vi "Automatic operation loop.vi"() -> ()   [LabVIEW 2016]
uses:
  <userlib>/LevyLab/Relay Box/Type_defs/Resistor--enum.ctl
  <userlib>/LevyLab/General AFM Lithography/subVIs/Global Variables.vi
panel:
  in  "Pulse Settings":T2={"Z Set point"=-0.03, "Set Resistance"=enum."0 ohms", "Wait between"=0, "Withdraw tip? 1"=TRUE, "Set Resistance 2"=enum."0 ohms", "Withdraw tip? 2"=TRUE} {"Z Set point" format="%#_6p"}
  in  "Repeat pulses (set V1 type to be repeating)":dbl=10.0
  in  "Stop Button":bool
  in  "Ready to apply pulses ?":bool
  out "Next T2":dbl=1000.0
  out "Next V2":dbl=10.0
  out "Next T1":dbl=600.0
  out "Next V1":dbl=-13.0
  out "error out":errorcluster
  in  "Cluster":T3={"V2 array"=[0.0, 1.0, 2.0, 3.0, 4.0, 5.0], "V1 array"=[0.0, 1.0, 2.0, 3.0, 4.0, 5.0], "T2 array"=[4.0], "T1 array"=[4.0]}
  in  "First voltage pulse":T4={"Vmin"=0.0, "Tmin"=200.0, "Vmax"=5.0, "Tmax"=600.0, "V Array"=[0.0, 1.0, 1.0, 1.0, 1.0], "T Array"=[10.0, 20.0, 40.0, 60.0, 80.0, 100.0, 200.0, 300.0, 400.0, 500.0, 600.0], "V step"=1.0, "T step"=100.0, "Constant V"=-13.0, "Constant T"=600.0, "V1 type"=enum."No-Sweep", "T1 type"=enum."No-Sweep"}
  out "V1 array":dbl[](array[numeric])=[-13.0]
  out "T1 array":dbl[](array[numeric])=[600.0]
  in  "vi path":path=path "C:/Program Files (x86)/National Instruments/LabVIEW 2016/user.lib/LevyLab/General AFM Lithography/Main_v4.vi"
  out "vi running ?":bool
  in  "error in (no error)":errorcluster
  in  "Objects to enable":string[](array[string])=["r3", "p0", "p3"]
  out "T2 array":dbl[](array[numeric])=[200.0, 300.0, 400.0, 500.0, 600.0, 700.0, 800.0, 900.0, 1000.0]
  out "V2 array":dbl[](array[numeric])=[10.0]
  out "Log":string="Log:\nPulse: (-13.00V, 600.00ms); wait 5000ms; Pulse: (10V, 200ms), wait 10000ms is DONE\nPulse: (-13.00V, 600.00ms); wait 5000ms; Pulse: (10V, 300ms), wait 10000ms is DONE\nPulse: (-13.00V, 600.00ms); wait 5000ms; Pulse: (10V, 400ms), wait 10000ms is DONE\nPulse: (-13.00V, 600.00ms); wait 5000ms; Pulse: (10V, 500ms), wait 10000ms is DONE\nPulse: (-13.00V, 600.00ms); wait 5000ms; Pulse: (10V, 600ms), wait 10000ms is DONE\nPulse: (-13.00V, 600.00ms); wait 5000ms; Pulse: (10V, 700ms), wait 10000ms is DONE\nPulse: (-13.00V, 600.00ms); wait 5000ms; Pulse: (10V, 800ms), wait 10000ms is DONE\nPulse: (-13.00V, 600.00ms); wait 5000ms; Pulse: (10V, 900ms), wait 10000ms is DONE\nPulse: (-13.00V, 600.00ms); wait 5000ms; Pulse: (10V, 1000ms), wait 10000ms is DONE\n"
  in  "Operation loop":T5(array[cluster])=[{"String"="p1", "Enum"=enum."Object", "Wait after"=0.0}, {"String"=".001", "Enum"=enum."Object", "Wait after"=0.0}, {"String"="p2", "Enum"=enum."Object", "Wait after"=500.0}, {"String"="", "Enum"=enum."Voltage pulse", "Wait after"=500.0}, {"String"="", "Enum"=enum."IV measurement", "Wait after"=500.0}]
  in  "Second voltage pulse":T6={"Vmin"=0.0, "Tmin"=200.0, "Vmax"=5.0, "Tmax"=1000.0, "V Array"=[0.0, 1.0, 1.0, 1.0, 1.0], "T Array"=[3.0, 3.0, 3.0, 3.0, 3.0], "V step"=1.0, "T step"=100.0, "Constant V"=10.0, "Constant T"=0.0, "V2 type"=enum."No-Sweep", "T2 type"=enum."Sweep (auto)"}
  # "Show the log of voltage parameter setting and corresponding IV record file name"
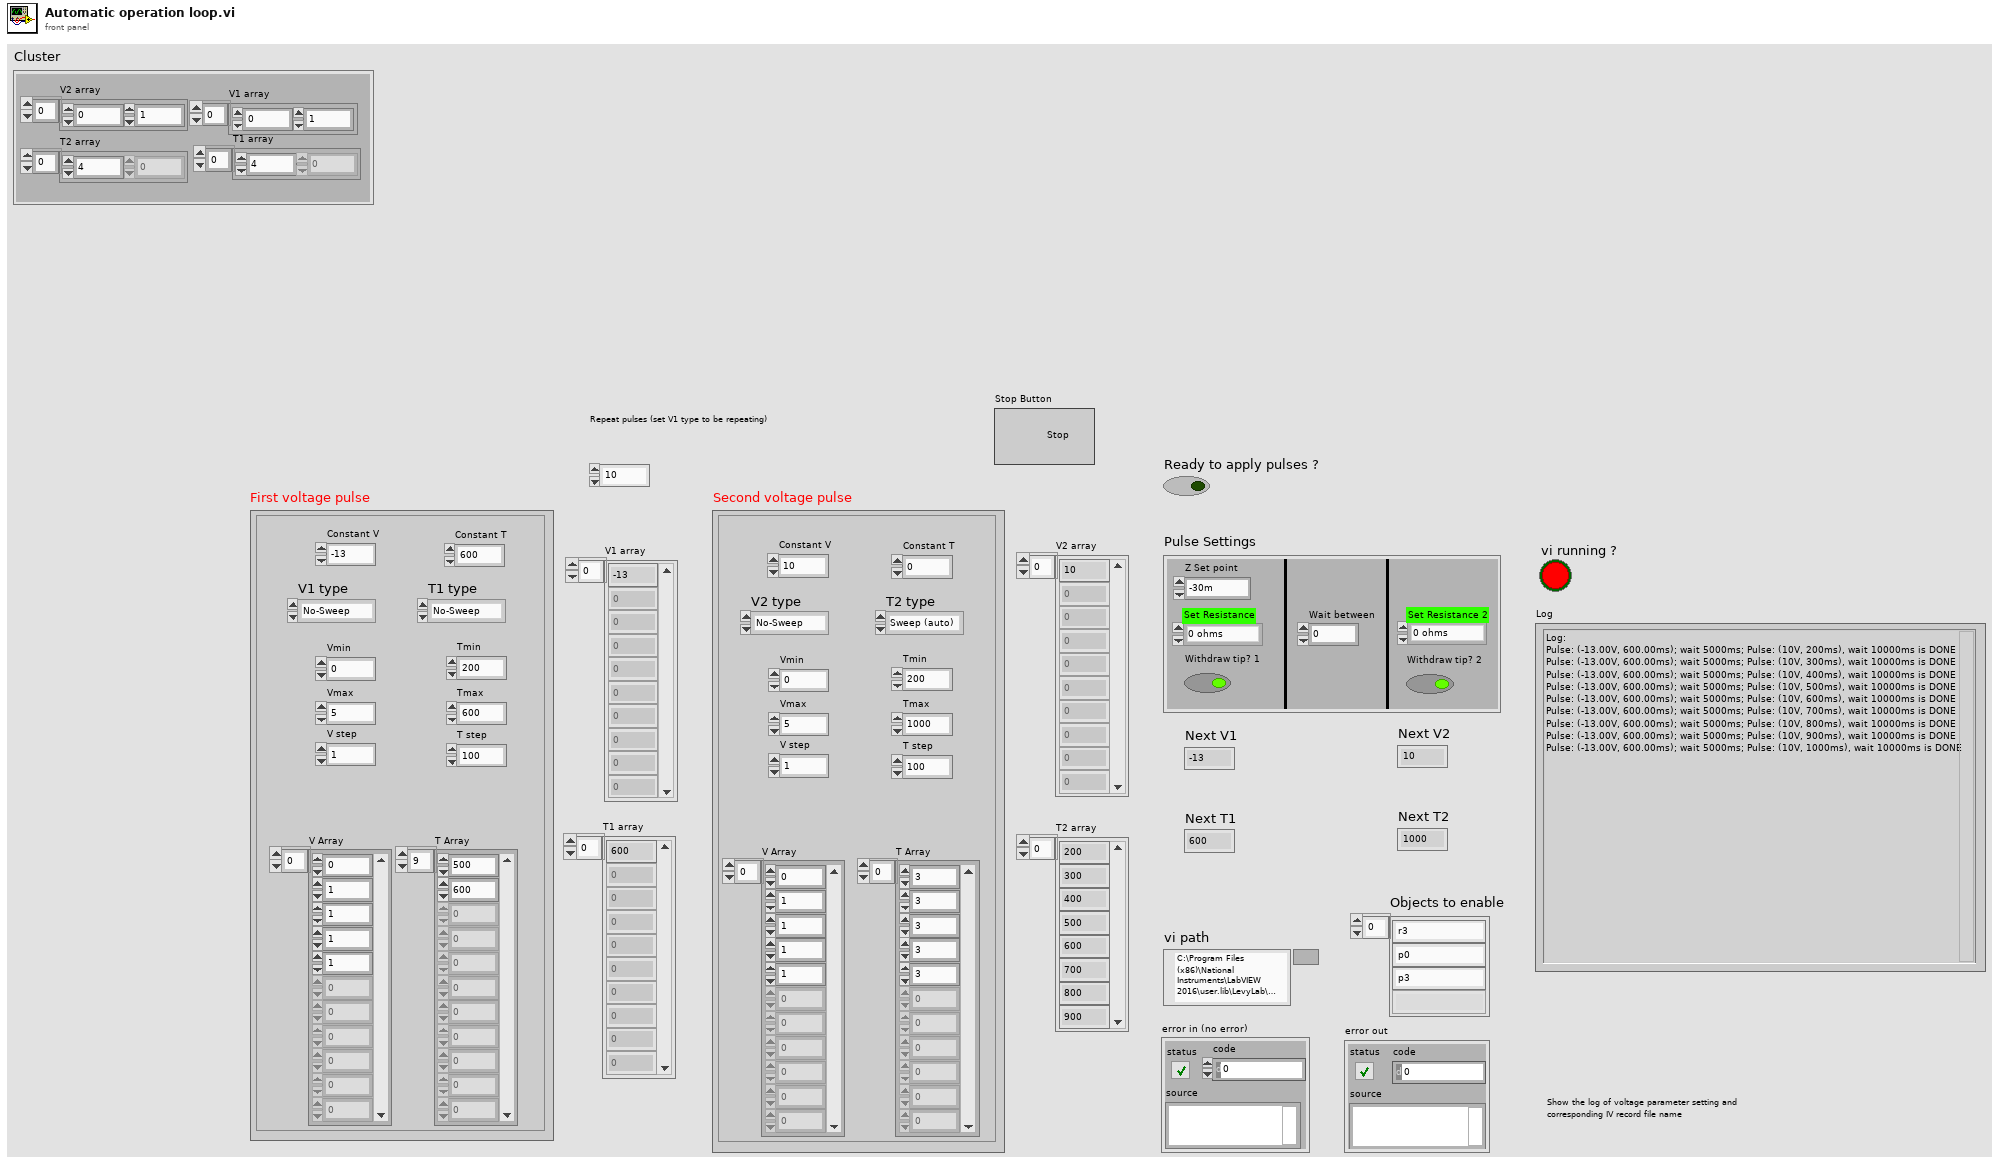
[diagram p1: front panel]
types:
  T1 = typedef "Resistor--enum.ctl" = enum16{"open", "discharge tip", "0 ohms", "100k ohm", "10M ohm", "1G ohm"}
  T2 = cluster{"Z Set point":dbl, "Set Resistance":T1, "Wait between":u32, "Withdraw tip? 1":bool, "Set Resistance 2":T1, "Withdraw tip? 2":bool}
  T3 = cluster{"V2 array":dbl[], "V1 array":dbl[], "T2 array":dbl[], "T1 array":dbl[]}
  T4 = cluster{"Vmin":dbl, "Tmin":dbl, "Vmax":dbl, "Tmax":dbl, "V Array":dbl[], "T Array":dbl[], "V step":dbl, "T step":dbl, "Constant V":dbl, "Constant T":dbl, "V1 type":enum16{"Repeating", "No-Sweep", "Sweep (manual)", "Sweep (auto)"}, "T1 type":enum16{"Repeating", "No-Sweep", "Sweep (manual)", "Sweep (auto)"}}
  T5 = cluster{"String":string, "Enum":enum16{"Object", "Voltage pulse", "IV measurement", "Change interpolation distance"}, "Wait after":dbl}[]
  T6 = cluster{"Vmin":dbl, "Tmin":dbl, "Vmax":dbl, "Tmax":dbl, "V Array":dbl[], "T Array":dbl[], "V step":dbl, "T step":dbl, "Constant V":dbl, "Constant T":dbl, "V2 type":enum16{"Repeating", "No-Sweep", "Sweep (manual)", "Sweep (auto)"}, "T2 type":enum16{"Repeating", "No-Sweep", "Sweep (manual)", "Sweep (auto)"}}
  T7 = enum16{"Object", "Voltage pulse", "IV measurement", "Change interpolation distance"}
  T8 = typedef "Funnel Properties - cluster.ctl" = cluster{"Enabled":bool, "Direction":u16, "Smooth Segments":dbl, "Bottom Segs.":dbl, "Speed (um/s)":T9, "Voltage (V)":T9, "Set Resistance":T1}
  T9 = typedef "Voltage - cluster.ctl" = cluster{"Schedule":T10, "Value":dbl, "Start Value":dbl, "End Value":dbl, "Min Value":dbl, "Max Value":dbl, "Duty Cycle (%)":dbl, "Signal Type":T11, "Cycle Number":dbl, "Phase (degrees)":dbl, "formula":string, "formula length (nm)":dbl, "formula resolution (nm)":dbl}
  T10 = typedef "Schedule - enum.ctl" = enum16{"Constant", "Ramp", "Fn. Generator", "Formula"}
  T11 = typedef "Signal Type - enum.ctl" = enum16{"Sine Wave", "Triangle Wave", "Square Wave", "Sawtooth Wave"}
  T12 = typedef "Path Properties - cluster.ctl" = cluster{"Enabled":bool, "Direction":u16, "Fill Orientation":u16, "Smooth Segments":dbl, "Fill Spacing":dbl, "Speed (um/s)":T9, "Voltage (V)":T9, "Set Resistance":T1}
  T13 = typedef "Rectangle Properties - cluster.ctl" = cluster{"Enabled":bool, "Direction":u16, "Fill Orientation":u16, "Fill Spacing":dbl, "Speed (um/s)":T9, "Voltage (V)":T9, "Set Resistance":T1}
  T14 = enum16{"Repeating", "No-Sweep", "Sweep (manual)", "Sweep (auto)"}
  T15 = cluster{"Set point":dbl, "Set Resistance":T1, "First pulse voltage":dbl, "First pulse time":u32, "Wait between":u32, "Second pulse voltage":dbl, "Second pulse time":u32, "Withdraw tip? 1":bool, "Set Resistance 2":T1, "Withdraw tip? 2":bool}
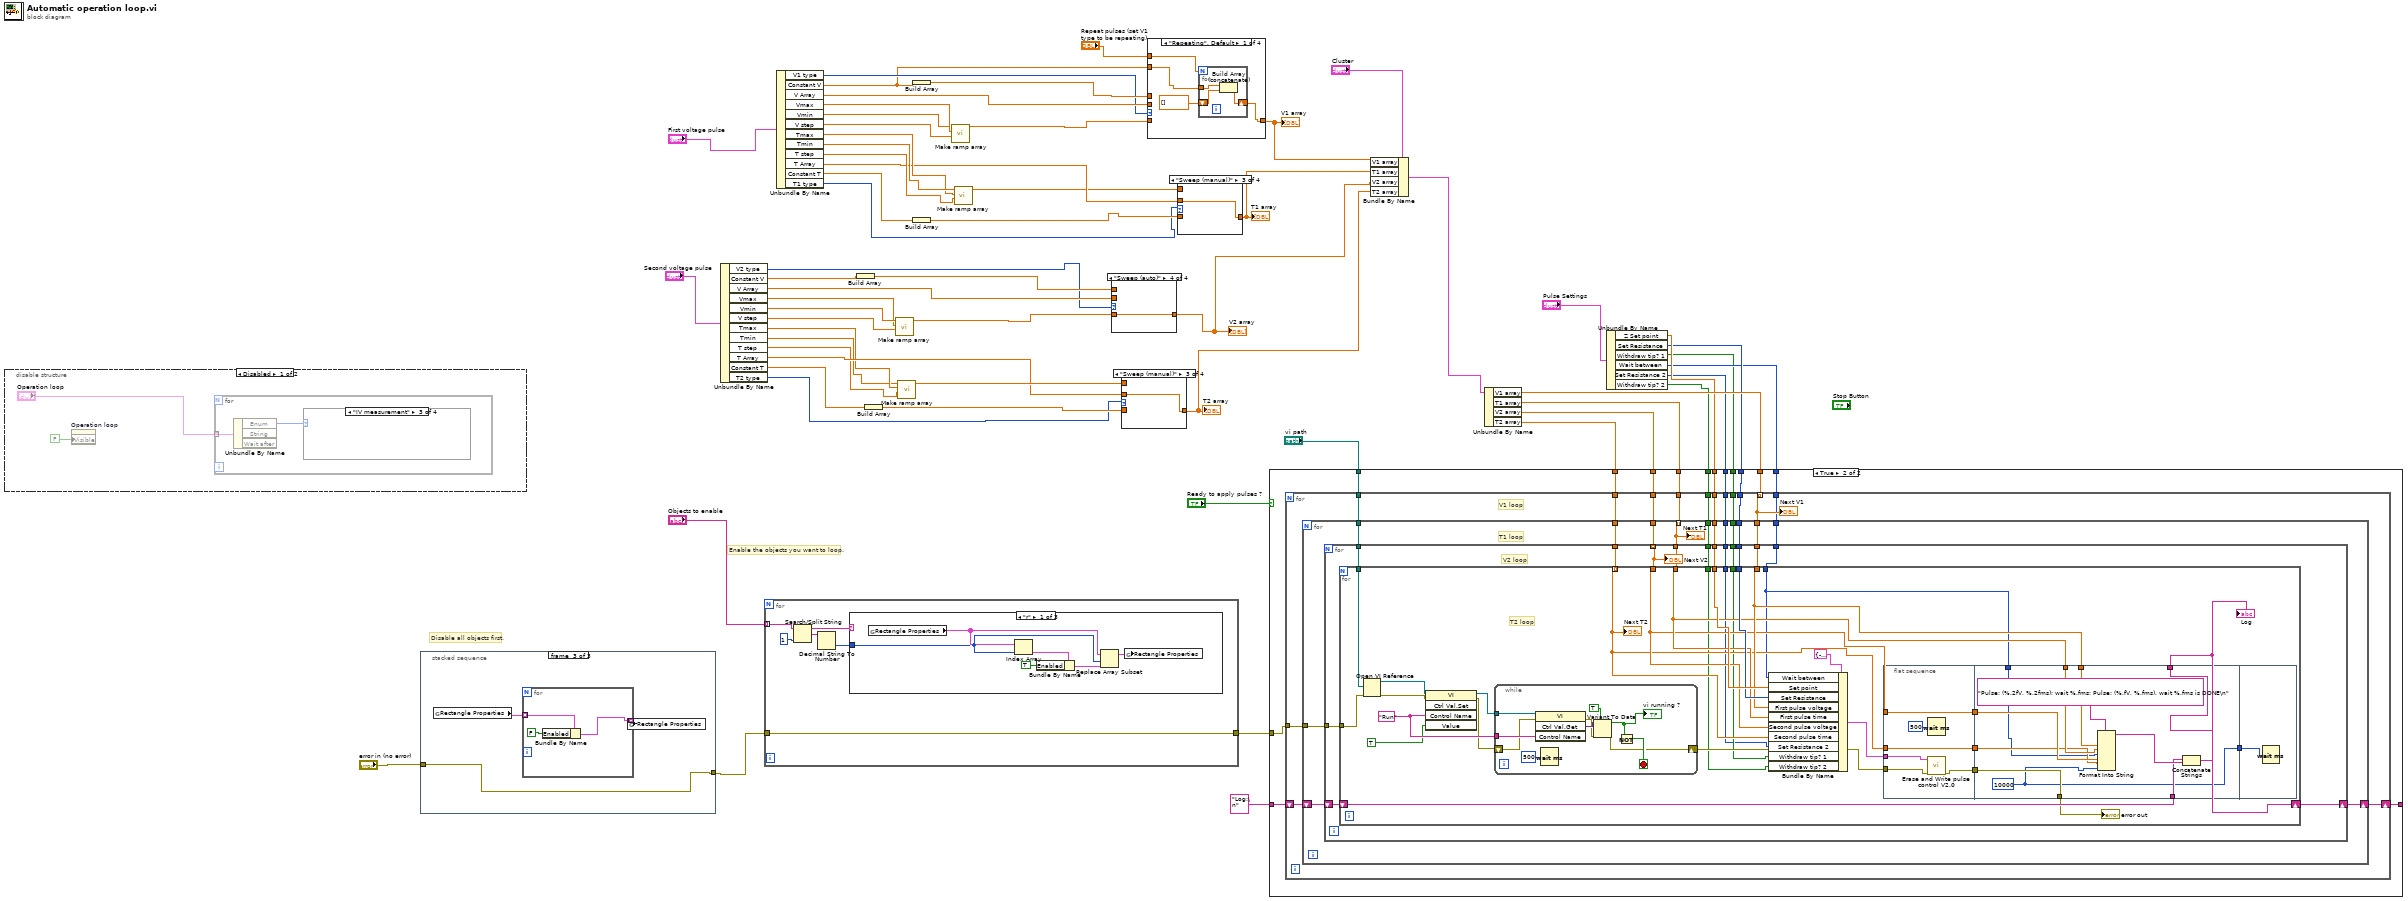
[diagram p0: block diagram]
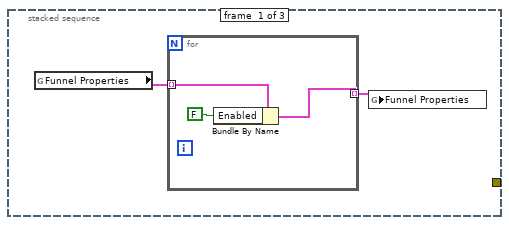
[diagram p19: hidden frame]
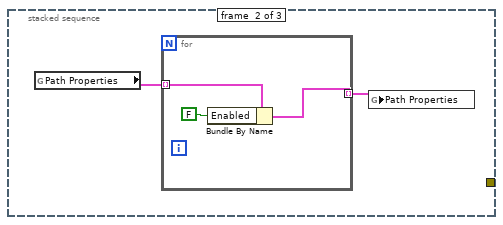
[diagram p20: hidden frame]
diagram:
  # "Disable all objects first."
  # "Enable the objects you want to loop."
  n1 = disable-structure shown="Disabled" {
    frame Disabled {
      n2 = property on="Operation loop" class="Arr (strict)"("Visible"=FALSE) -> ()  [unwired: 2 in, 2 out]
      n3 = for {
        tunnel: "Operation loop" -> [w63] mode=indexing
        n4 = Unbundle By Name(w63) -> ("Enum"=w62:T7)  [unwired: 2 out]
        n5 = case shown="\"IV measurement\"" w62 {
          frame "Object", Default {
            # "Enable the object in litho.vi and run the vi"
          }
          frame "Voltage pulse" {
          }
          frame "IV measurement" {
          }
          frame "Change interpolation distance" {
          }
        }
      }
    }
    frame Enabled {
    }
  }
  n6 = stacked-sequence {
    tunnel: "error in (no error)" -> [_ _ w74]
    tunnel: [_ _ w74] -> w56
    frame #0 {
      n7 = global read "Global Variables.vi" "Funnel Properties"() -> (w64:T8[])
      n8 = for {
        tunnel: w64 -> [w67] mode=indexing
        tunnel: [w66] -> w65 mode=indexing
        n9 = Bundle By Name(cluster=w67, "Enabled"=FALSE) -> (w66:T8)
      }
      n10 = global write "Global Variables.vi" "Funnel Properties"(w65) -> ()
    }
    frame #1 {
      n11 = global read "Global Variables.vi" "Path Properties"() -> (w69:T12[])
      n12 = for {
        tunnel: w69 -> [w72] mode=indexing
        tunnel: [w71] -> w70 mode=indexing
        n13 = Bundle By Name(cluster=w72, "Enabled"=FALSE) -> (w71:T12)
      }
      n14 = global write "Global Variables.vi" "Path Properties"(w70) -> ()
    }
    frame #2 {
      n15 = global read "Global Variables.vi" "Rectangle Properties"() -> (w75:T13[])
      n16 = for {
        tunnel: w75 -> [w78] mode=indexing
        tunnel: [w77] -> w76 mode=indexing
        n17 = Bundle By Name(cluster=w78, "Enabled"=FALSE) -> (w77:T13)
      }
      n18 = global write "Global Variables.vi" "Rectangle Properties"(w76) -> ()
    }
  }
  n19 = Unbundle By Name("Second voltage pulse") -> ("V2 type"=w20:T14, "Constant V"=w23:dbl, "V Array"=w31:dbl[], "Vmax"=w28:dbl, "Vmin"=w29:dbl, "V step"=w27:dbl, "Tmax"=w26:dbl, "Tmin"=w25:dbl, "T step"=w24:dbl, "T Array"=w34:dbl[], "Constant T"=w22:dbl, "T2 type"=w19:T14)
  n20 = for {
    tunnel: "Objects to enable" -> [w81] mode=indexing
    tunnel: [w80] -> w58
    tunnel: w56 -> [w80]
    n21 = Search/Split String(string=w81, offset (0)=1) -> (substring before match=w83:string, match + rest of string=w84:string)  [unwired: 1 in, 1 out]
    n22 = Decimal String To Number(string=w84) -> (number=w82:i32)  [unwired: 2 in, 1 out]
    n23 = case shown="\"r\"" w83 {
      tunnel: w82 -> [w86 w92 w98]
      frame "r" {
        n24 = global read "Global Variables.vi" "Rectangle Properties"() -> (w90:T13[])
        n25 = Index Array(array=w90, index=w86) -> (element=w87:T13)
        n26 = Bundle By Name(cluster=w87, "Enabled"=TRUE) -> (w88:T13)
        n27 = Replace Array Subset(array=w90, new element=w88, index=w86) -> (w91:T13[])
        n28 = global write "Global Variables.vi" "Rectangle Properties"(w91) -> ()
      }
      frame "p", Default {
        n29 = global read "Global Variables.vi" "Path Properties"() -> (w96:T12[])
        n30 = Index Array(array=w96, index=w92) -> (element=w93:T12)
        n31 = Bundle By Name(cluster=w93, "Enabled"=TRUE) -> (w94:T12)
        n32 = Replace Array Subset(array=w96, new element=w94, index=w92) -> (w97:T12[])
        n33 = global write "Global Variables.vi" "Path Properties"(w97) -> ()
      }
      frame "f" {
        n34 = global read "Global Variables.vi" "Funnel Properties"() -> (w102:T8[])
        n35 = Index Array(array=w102, index=w98) -> (element=w99:T8)
        n36 = Bundle By Name(cluster=w99, "Enabled"=TRUE) -> (w100:T8)
        n37 = Replace Array Subset(array=w102, new element=w100, index=w98) -> (w103:T8[])
        n38 = global write "Global Variables.vi" "Funnel Properties"(w103) -> ()
      }
    }
  }
  n39 = Unbundle By Name("First voltage pulse") -> ("V1 type"=w18:T14, "Constant V"=w9:dbl, "V Array"=w40:dbl[], "Vmax"=w44:dbl, "Vmin"=w43:dbl, "V step"=w45:dbl, "Tmax"=w46:dbl, "Tmin"=w47:dbl, "T step"=w48:dbl, "T Array"=w37:dbl[], "Constant T"=w49:dbl, "T1 type"=w17:T14)
  n40 = Build Array(w23) -> (w32:dbl[])
  n41 = Build Array(w22) -> (w33:dbl[])
  n42 = call "Make ramp array.vi"("step"=w27, "end"=w28, "start"=w29) -> ("Ramp Array"=w30:dbl[])  [unwired: 8 in]
  n43 = call "Make ramp array.vi"("step"=w24, "end"=w26, "start"=w25) -> ("Ramp Array"=w35:dbl[])  [unwired: 8 in]
  n44 = Build Array(w9) -> (w39:dbl[])
  n45 = Build Array(w49) -> (w38:dbl[])
  n46 = call "Make ramp array.vi"("step"=w45, "end"=w44, "start"=w43) -> ("Ramp Array"=w41:dbl[])  [unwired: 8 in]
  n47 = call "Make ramp array.vi"("step"=w48, "end"=w46, "start"=w47) -> ("Ramp Array"=w36:dbl[])  [unwired: 8 in]
  n48 = case shown="\"Sweep (auto)\"" w20 {
    tunnel: [_ w104 w105 w106] -> w51
    tunnel: w30 -> [_ _ _ w106]
    tunnel: w31 -> [_ _ w105 _]
    tunnel: w32 -> [_ w104 _ _]
    frame "Repeating", Default {
    }
    frame "No-Sweep" {
    }
    frame "Sweep (manual)" {
    }
    frame "Sweep (auto)" {
    }
  }
  "V2 array" <- w51
  n49 = case shown="\"Sweep (manual)\"" w19 {
    tunnel: [_ w107 w108 w109] -> w50
    tunnel: w34 -> [_ _ w108 _]
    tunnel: w33 -> [_ w107 _ _]
    tunnel: w35 -> [_ _ _ w109]
    frame "Repeating", Default {
    }
    frame "No-Sweep" {
    }
    frame "Sweep (manual)" {
    }
    frame "Sweep (auto)" {
    }
  }
  "T2 array" <- w50
  n50 = case shown="\"Repeating\", Default" w18 {
    tunnel: [w111 w117 w118 w119] -> w53
    tunnel: w41 -> [_ _ _ w119]
    tunnel: w40 -> [_ _ w118 _]
    tunnel: w39 -> [_ w117 _ _]
    tunnel: w9 -> [w113 _ _ _]
    tunnel: "Repeat pulses (set V1 type to be repeating)" -> [w110 _ _ _]
    frame "Repeating", Default {
      n51 = for {
        N: w110 -> [_]
        tunnel: w113 -> [w114]
        shift-right: [w115] -> w111
        shift-left: dbl[] [] ("Ramp Array") -> [w116]
        n52 = Build Array (concatenate)(w114, w116) -> (w115:dbl[])
      }
    }
    frame "No-Sweep" {
    }
    frame "Sweep (manual)" {
    }
    frame "Sweep (auto)" {
    }
  }
  "V1 array" <- w53
  n53 = case shown="\"Sweep (manual)\"" w17 {
    tunnel: [_ w120 w121 w122] -> w52
    tunnel: w37 -> [_ _ w121 _]
    tunnel: w38 -> [_ w120 _ _]
    tunnel: w36 -> [_ _ _ w122]
    frame "Repeating", Default {
    }
    frame "No-Sweep" {
    }
    frame "Sweep (manual)" {
    }
    frame "Sweep (auto)" {
    }
  }
  "T1 array" <- w52
  n54 = Bundle By Name(cluster="Cluster", "V1 array"=w53, "T1 array"=w52, "V2 array"=w51, "T2 array"=w50) -> (w10:T3)
  n55 = Unbundle By Name(w10) -> ("V1 array"=w16:dbl[], "T1 array"=w15:dbl[], "V2 array"=w14:dbl[], "T2 array"=w13:dbl[])
  n56 = Unbundle By Name("Pulse Settings") -> ("Z Set point"=w6:dbl, "Set Resistance"=w5:T1, "Withdraw tip? 1"=w3:bool, "Wait between"=w4:u32, "Set Resistance 2"=w1:T1, "Withdraw tip? 2"=w2:bool)
  n57 = case shown="True" "Ready to apply pulses ?" {
    tunnel: w58 -> [_ w136]
    tunnel: "vi path" -> [_ w135]
    tunnel: w16 -> [_ w134]
    tunnel: w15 -> [_ w133]
    tunnel: w14 -> [_ w132]
    tunnel: w13 -> [_ w131]
    tunnel: w6 -> [_ w130]
    tunnel: w5 -> [_ w129]
    tunnel: "Log:\n" ("format string") -> [_ w128]
    tunnel: [_ w127] -> _
    tunnel: w4 -> [_ w126]
    tunnel: w3 -> [_ w125]
    tunnel: w2 -> [_ w124]
    tunnel: w1 -> [_ w123]
    frame False {
    }
    frame True {
      n58 = for {
        tunnel: w136 -> [w150]
        tunnel: w135 -> [w149]
        tunnel: w134 -> [w148] mode=indexing
        tunnel: w133 -> [w147]
        tunnel: w132 -> [w146]
        tunnel: w131 -> [w145]
        tunnel: w130 -> [w144]
        tunnel: w129 -> [w143]
        shift-right: [w141] -> w127
        shift-left: w128 -> [w142]
        tunnel: w126 -> [w140]
        tunnel: w125 -> [w139]
        tunnel: w124 -> [w138]
        tunnel: w123 -> [w137]
        # "V1 loop"
        n59 = for {
          tunnel: w150 -> [w164]
          tunnel: w149 -> [w163]
          tunnel: w148 -> [w162]
          tunnel: w147 -> [w161] mode=indexing
          tunnel: w146 -> [w160]
          tunnel: w145 -> [w159]
          tunnel: w144 -> [w158]
          tunnel: w143 -> [w157]
          shift-right: [w155] -> w141
          shift-left: w142 -> [w156]
          tunnel: w140 -> [w154]
          tunnel: w139 -> [w153]
          tunnel: w138 -> [w152]
          tunnel: w137 -> [w151]
          # "T1 loop"
          n60 = for {
            tunnel: w164 -> [w178]
            tunnel: w163 -> [w177]
            tunnel: w162 -> [w176]
            tunnel: w161 -> [w175]
            tunnel: w160 -> [w174] mode=indexing
            tunnel: w159 -> [w173]
            tunnel: w158 -> [w172]
            tunnel: w157 -> [w171]
            shift-right: [w169] -> w155
            shift-left: w156 -> [w170]
            tunnel: w154 -> [w168]
            tunnel: w153 -> [w167]
            tunnel: w152 -> [w166]
            tunnel: w151 -> [w165]
            # "V2 loop"
            n61 = for {
              tunnel: w178 -> [w200]
              tunnel: w177 -> [w199]
              tunnel: w176 -> [w194]
              tunnel: w175 -> [w193]
              tunnel: w174 -> [w192]
              tunnel: w173 -> [w191] mode=indexing
              tunnel: w172 -> [w196]
              tunnel: w171 -> [w195]
              shift-right: [w183] -> w169
              shift-left: w170 -> [w190]
              tunnel: w168 -> [w185]
              tunnel: w167 -> [w181]
              tunnel: w166 -> [w180]
              tunnel: w165 -> [w179]
              w206 = "Run" ("Control Name")
              # "T2 loop"
              n62 = Open VI Reference(vi path=w199, error in (no error)=w200) -> (vi reference=w203:refnum<vi>, error out=w202:errorcluster)  [unwired: 4 in]
              n63 = invoke class="VI" method="Ctrl Val.Set"(reference=w203, error in=w202, "Control Name"=w206, "Value"=TRUE) -> (reference out=w205:refnum<vi>, error out=w201:errorcluster)  [unwired: 1 in, 3 out]
              n64 = while {
                tunnel: w205 -> [w234]
                tunnel: w206 -> [w233]
                shift-right: [w229] -> w197
                shift-left: w201 -> [w227]
                stop <- w230 stop-if-true
                n65 = invoke class="VI" method="Ctrl Val.Get"(reference=w234, error in=w227, "Control Name"=w233) -> (error out=w226:errorcluster, "Get Control Value Variant"=w232:variant)  [unwired: 1 in, 2 out]
                n66 = Wait (ms)(milliseconds to wait=u32 500) -> ()  [unwired: 1 out]
                n67 = Variant To Data(error in=w226, type=TRUE, Variant=w232) -> (data=w225:bool, error out=w229:errorcluster)
                "vi running ?" <- w225
                n68 = Not(x=w225) -> (.not. x?=w230:bool)
              }
              n69 = Bundle By Name(cluster=T15 {"Set point"=-0.03, "Set Resistance"=enum."0 ohms", "First pulse voltage"=-10.0, "First pulse time"=10, "Wait between"=0, "Second pulse voltage"=0.0, "Second pulse time"=500, "Withdraw tip? 1"=TRUE, "Set Resistance 2"=enum."0 ohms", "Withdraw tip? 2"=TRUE} ("Pulse Settings"), "Wait between"=w185, "Set point"=w196, "Set Resistance"=w195, "First pulse voltage"=w194, "First pulse time"=w193, "Second pulse voltage"=w192, "Second pulse time"=w191, "Set Resistance 2"=w179, "Withdraw tip? 1"=w181, "Withdraw tip? 2"=w180) -> (w198:T15)
              n70 = flat-sequence {
                tunnel: w191 -> [w211]
                tunnel: w192 -> [w212]
                tunnel: w197 -> [w208]
                tunnel: w198 -> [w209]
                tunnel: [w212] -> w189
                tunnel: [w211] -> w188
                tunnel: [w207] -> w187
                tunnel: w194 -> [w223]
                tunnel: w193 -> [w222]
                tunnel: w190 -> [w217]
                tunnel: w189 -> [w221]
                tunnel: w188 -> [w220]
                tunnel: [w213] -> w183
                tunnel: w187 -> [w216]
                tunnel: [w216] -> w186
                tunnel: w185 -> [w215]
                tunnel: [w214] -> w184
                tunnel: w184 -> [w224]
                frame #0 {
                  n71 = call "Erase and Write pulse control V2.0.vi"("error in"=w208, "Pulse Settings"=w209) -> ("error out"=w207:errorcluster)  [unwired: 9 in]
                  n72 = Wait (ms)(milliseconds to wait=u32 500) -> ()  [unwired: 1 out]
                }
                frame #1 {
                  w214 = u32 10000 ("milliseconds to wait")
                  n73 = Format Into String(format string="Pulse: (%.2fV, %.2fms); wait %.fms; Pulse: (%.fV, %.fms), wait %.fms is DONE\n", w223, w222, w215, w221, w220, w214) -> (resulting string=w218:string)  [unwired: 2 in, 1 out]
                  n74 = Concatenate Strings(w217, w218) -> (w213:string)
                }
                frame #2 {
                  n75 = Wait (ms)(milliseconds to wait=w224) -> ()  [unwired: 1 out]
                }
              }
              "Next T2" <- w191
              "Log" <- w183
              "error out" <- w186
            }
            "Next V2" <- w174
          }
          "Next T1" <- w161
        }
        "Next V1" <- w148
      }
    }
  }
